vi "Motor Move XYZ-AOL Zstack.vi"(8 "error in (no error)":errorcluster, 9 "Zplane in":i32, 10 "AOL_Globals":T1={"Imaging Protocol"=enum."AOL Z-Stack", "Number of POI"=0, "Number of Miniscans"=0, "Number of Trials"=0, "Number of Cycles "=0, "# Averaged Frames"=0, "Laser power (%)"=0, "Pockels (V)"=0.0, "Acquisition Length (sec)"=0.0, "Fill time (us)"=0.0, "POI Dwell time (us)"=0.0, "Miniscan Dwell time per pixel (us)"=0.0, "PMT 1"=0.0, "PMT 2"=0.0, "Back Apperture (mA)"=200.0, "Frame Size"=0, "Center Frequency"=0.0, "Field of View (um)"=175.0, "Field of View (norm)"=0.0, "DwellTime (us)"=0.0, "Ref Dwell Time (us)"=0.0, "Wavelength (nm)"=0.0, "Zoom"=0.0, "AOL Z"=0.0, "AOL Mode"=enum."Raster", "GridXY"=0.0, "GridZ"=0.0, "TriggerPeriod (sec)"=0.0, "Number of Pixels in Miniscan"=0, "Experiment folder path"=path "", "X centre"=0.0, "Y centre"=0.0, "Angle (degrees)"=0.0, "Angle Xs (degrees)"=0.0, "Angle Ys (degrees)"=0.0, "Plane Mode"=0, "Threshold"=[], "Regenerate Chirps"=FALSE, "Rectangle ROI length (pixels)"=0, "Rectangle ROI height (pixels)"=0, "AOD fill"=4900, "StartupDelay"=0, "Samples Wait after Trigger"=5080, "Slip Cycle"=600000, "Add Cycle"=TRUE, "Functional Mode"=enum."Point", "Z Start"=0.0, "Z Stop"=0.0, "# Planes"=0, "Total Pixels"=0, "Variable Miniscan Pixels"=[], "Use Variable Length"=FALSE, "Use Variable Resolution"=FALSE, "Laser power (%) at Z Start"=0, "Laser power (%) at Z Stop"=0, "Ref Z Step"=0} {"Angle Ys (degrees)" format="%#.6g"; "Angle Xs (degrees)" format="%#.6g"; "Plane Mode" items=["XY Plane", "XZ Plane", "YZ Plane", "arbitraryplane"]; "Frame Size" items=["100X100"=100, "128X128"=128, "200X200"=200, "256X256"=256, "512X512"=512, "1024x1024"=1024, "2048x2048"=2048]; "Back Apperture (mA)" format="%#.6g"; "Pockels (V)" format="%#.6g"; "PMT 2" format="%#.6g"; "PMT 1" format="%#.6g"; "Angle (degrees)" format="%#.6g"; "POI Dwell time (us)" format="%#.6g"}) -> (0 "error out":errorcluster)   [LabVIEW 2020]
uses:
  Typedefs/Controls/AOL_Globals.ctl
  Typedefs/Imaging Protocols enum.ctl
  Typedefs/Frame Size.ctl
  Typedefs/AOL modes.ctl
  Typedefs/Plane Mode.ctl
  Typedefs/Functional Mode.ctl
  Typedefs/HW config states enum.ctl
  Typedefs/Read Write Enum.ctl
  Global Variables/General Globals.vi
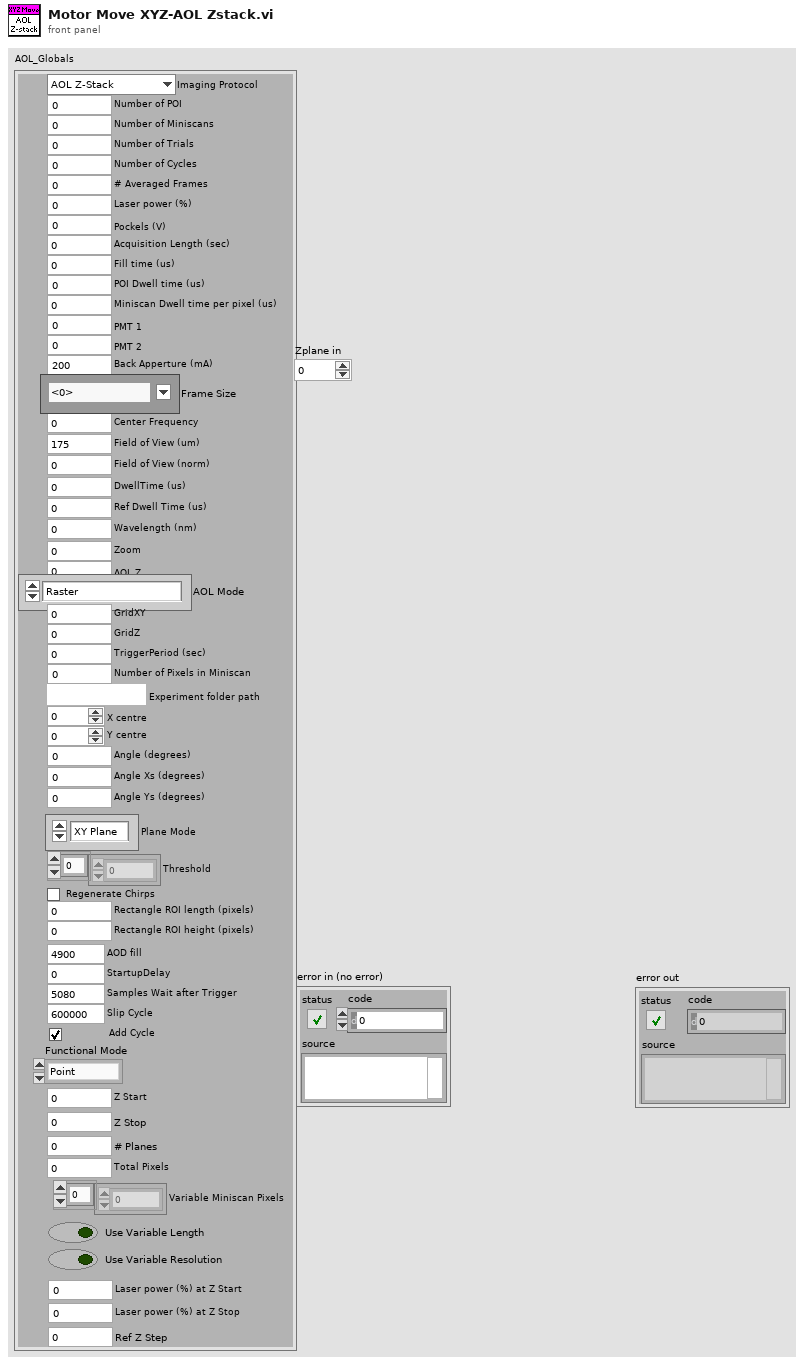
[diagram p1: front panel]
types:
  T1 = typedef "AOL_Globals.ctl" = cluster{"Imaging Protocol":T2, "Number of POI":u16, "Number of Miniscans":u16, "Number of Trials":u16, "Number of Cycles ":u64, "# Averaged Frames":u16, "Laser power (%)":u8, "Pockels (V)":dbl, "Acquisition Length (sec)":dbl, "Fill time (us)":dbl, "POI Dwell time (us)":dbl, "Miniscan Dwell time per pixel (us)":dbl, "PMT 1":dbl, "PMT 2":dbl, "Back Apperture (mA)":dbl, "Frame Size":T3, "Center Frequency":dbl, "Field of View (um)":dbl, "Field of View (norm)":dbl, "DwellTime (us)":dbl, "Ref Dwell Time (us)":dbl, "Wavelength (nm)":dbl, "Zoom":dbl, "AOL Z":dbl, "AOL Mode":T4, "GridXY":dbl, "GridZ":dbl, "TriggerPeriod (sec)":dbl, "Number of Pixels in Miniscan":u16, "Experiment folder path":path, "X centre":dbl, "Y centre":dbl, "Angle (degrees)":dbl, "Angle Xs (degrees)":dbl, "Angle Ys (degrees)":dbl, "Plane Mode":T5, "Threshold":u16[], "Regenerate Chirps":bool, "Rectangle ROI length (pixels)":u16, "Rectangle ROI height (pixels)":u16, "AOD fill":u16, "StartupDelay":i32, "Samples Wait after Trigger":u16, "Slip Cycle":u32, "Add Cycle":bool, "Functional Mode":T6, "Z Start":dbl, "Z Stop":dbl, "# Planes":i32, "Total Pixels":i32, "Variable Miniscan Pixels":u16[], "Use Variable Length":bool, "Use Variable Resolution":bool, "Laser power (%) at Z Start":u8, "Laser power (%) at Z Stop":u8, "Ref Z Step":i8}
  T2 = typedef "Imaging Protocols enum.ctl" = enum16{"AOL Z-Stack", "Motor Z Stack", "Parameter Sweep", "Functional Acquisition", "Single Plane Acquisition", "Volume Acquisition", "Live Imaging", "Live Plane Imaging", "Live Volume Imaging"}
  T3 = typedef "Frame Size.ctl" = u16
  T4 = typedef "AOL modes.ctl" = enum16{"Raster", "Structural", "Pointing", "Mini Scan", "Alignment"}
  T5 = typedef "Plane Mode.ctl" = u16
  T6 = typedef "Functional Mode.ctl" = enum16{"Point", "Line", "Patch", "Plane", "Volume"}
  T7 = typedef "HW config states enum.ctl" = enum16{"Load from file", "Save to file", "Save backup", "Write all", "Read all", "Write XY stage settings", "Write DAQ FPGA settings", "Write Control FPGA settings", "Write Phys Channels", "Write System Config", "Write HW Config", "Save System Config", "Save HW Config", "Clear", "Compare from file"}
  T8 = typedef "Read Write Enum.ctl" = enum16{"Read", "Write"}
  T9 = typedef "Hardware Configuration settings.ctl" = cluster{"Dev. PC":bool, "Swap XY on stage":bool, "No of AOD":u8, "MC Supported":bool, "Axial MC":bool, "Computer MAC address":string, "Externalise Triggers":bool, "Trigger HW config":T10, "DAQmx Chan":T11, "XYZ Stage Control Config":T12, "XY stage available":bool, "XY Comms Config Cluster":T13, "Y stage available":bool, "Y Comms Config Cluster":T13, "Z stage available":bool, "Z Comms Config Cluster ":T13, "Encoder available":bool, "Encoder":T15, "VidRec available":bool, "Cam VidRec":T16, "Laser Power Control HW config":T17, "Laser 1 available":bool, "Laser 1 config cluster":T18, "Prechirper 1 available":bool, "Prechirper 1 config cluster":T19, "Control system.FPGA available?":bool, "Control Sys. HW config":T20, "DAQ FPGA HW Config":T21, "PMT Control Voltage Limits":T25}
  T10 = typedef "Triggers HW config.ctl" = cluster{"Available Device List":i32, "Device Address":string}
  T11 = typedef "DAQmx physical channels cluster.ctl" = cluster{"Pockels AO":tag, "Hard shutter AO":tag, "PMT AOs":tag, "Galvo AOs":tag, "Power meter AI":tag}
  T12 = typedef "XYZControlConfig.ctl" = enum16{"None", "XYZ", "XY-Z", "X-Y-Z", "Z"}
  T13 = typedef "Peripherals comms config cluster.ctl" = cluster{"Name":string, "Device Address":string, "Port ":u16, "Baudrate":i32, "Comms Type":T14}
  T14 = typedef "Comms Type.ctl" = enum16{"GPIB-IEEE488", "Serial-RS232", "Serial-RS485", "Serial-RS422", "Serial-USB", "Ethernet-TCP/IP", "Ethernet-UDP"}
  T15 = typedef "Encoder config cluster.ctl" = cluster{"IP address":string, "Port":u16, "Wheel radius (cm)":dbl, "Encoder Trigger":tag}
  T16 = typedef "Cam VidRec HW config setup cluster.ctl" = cluster{"DO flag-Video record":tag, "DO flag-Trial start":tag}
  T17 = typedef "Laser Power Control HW config.ctl" = cluster{"Laser Power Control":string, "Laser Power Modulation Control":enum16{"NI", "FPGA"}}
  T18 = typedef "Laser 1 config cluster.ctl" = cluster{"COM port":refnum<visa-resource-name>, "Baud Rate":i32, "Type":string}
  T19 = typedef "PreChirper 1 config cluster.ctl" = cluster{"Type":string, "Baud Rate":i32, "COM port":refnum<visa-resource-name>}
  T20 = typedef "Control Sys HW config cluster.ctl" = cluster{"Control system.FPGA Type":enum16{"Virtex 5", "Virtex 7"}, "Control system.Network adapter name":string, "Control system.MAC address":string, "Control system.Ethernet Port":u32, "Control system.Ethernet Port Opened":bool}
  T21 = typedef "DAQ FPGA HW config cluster.ctl" = cluster{"FGPA Ref":T22, "Target":T23, "input card type":T24}
  T22 = typedef "FPGA Ref.ctl" = refnum<k20>
  T23 = typedef "nirio_resource_hc.ctl" = tag
  T24 = typedef "FPGA input type AC-DC.ctl" = enum16{"AC Card", "DC Card"}
  T25 = typedef "PMT Control Voltage limits.ctl" = cluster{"Lower Limit":dbl, "Upper Limit":dbl}
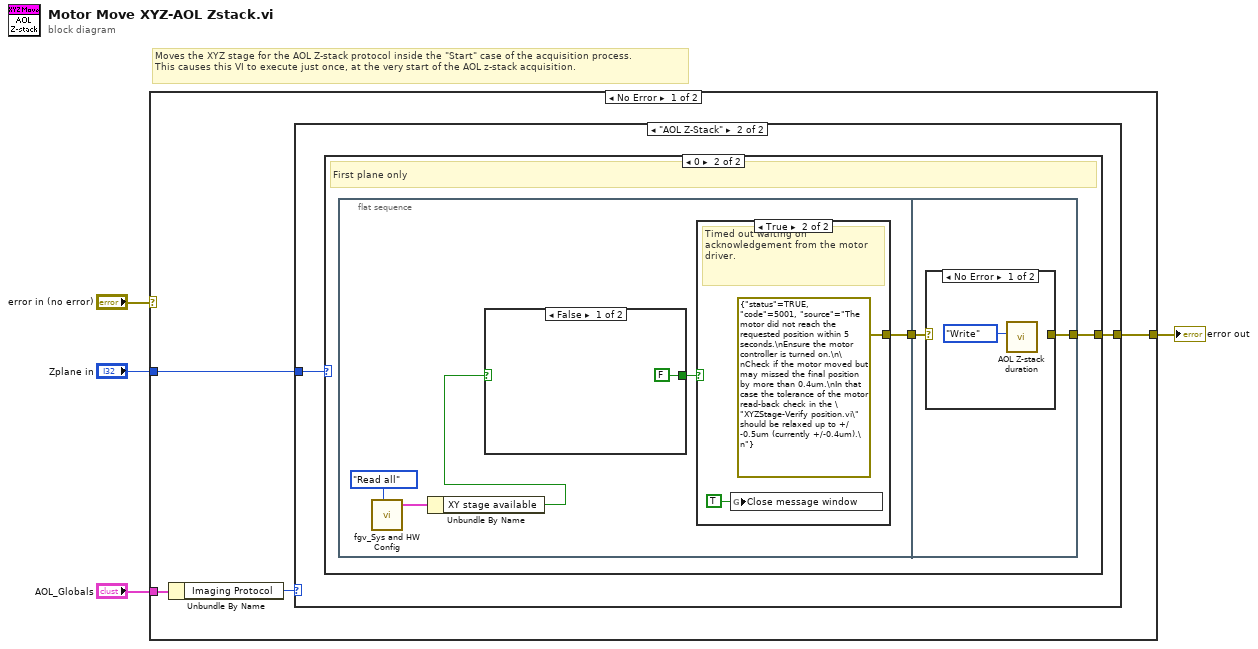
[diagram p0: block diagram]
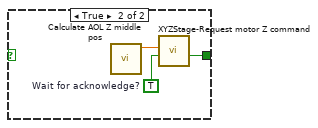
[diagram p4: hidden frame]
diagram:
  # "Moves the XYZ stage for the AOL Z-stack protocol inside the \"Start\" case of the acquisition process.\nThis causes this VI to execute just once, at the very start of the AOL z-stack acquisition."
  n1 = case shown="No Error" "error in (no error)" {
    selector: "error in (no error)" -> [_ w28]
    tunnel: [w5 w28] -> w3
    tunnel: "AOL_Globals" -> [w7 _]
    tunnel: "Zplane in" -> [w6 _]
    frame No Error {
      n2 = Unbundle By Name(w7) -> ("Imaging Protocol"=w8:T2)
      n3 = case shown="\"AOL Z-Stack\"" w8 {
        tunnel: w6 -> [_ w10]
        tunnel: [_ w9] -> w5
        frame Default {
        }
        frame "AOL Z-Stack" {
          n4 = case shown="0" w10 {
            tunnel: [_ w11] -> w9
            frame Default {
            }
            frame 0 {
              # "First plane only"
              n5 = flat-sequence {
                tunnel: [w16] -> w12
                tunnel: w12 -> [w25]
                tunnel: [w24] -> w11
                frame #0 {
                  n6 = call "fgv_Sys and HW Config.vi"("Function"=HW_config_states_enum."Read all") -> ("Hardware Configuration OUT"=w15:T9)  [unwired: 8 in, 2 out]
                  n7 = Unbundle By Name(w15) -> ("XY stage available"=w13:bool)
                  n8 = case shown="False" w13 {
                    tunnel: [FALSE ("Timed out while waiting for acknowledgement") w19] -> w17
                    frame False {
                    }
                    frame True {
                      w20 = TRUE  # Wait for acknowledge?
                      n9 = call "Calculate AOL Z middle pos.vi"() -> ("AOL Z-stack middle position"=w21:dbl)  [unwired: 11 in]
                      n10 = call "XYZStage-Request motor Z command.vi"("Wait for acknowledge?"=w20, "Motor Z"=w21) -> ("Timed out while waiting for acknowledgement"=w19:bool)  [unwired: 7 in, 2 out]
                    }
                  }
                  n11 = case shown="True" w17 {
                    tunnel: [_ errorcluster {"status"=TRUE, "code"=5001, "source"="The motor did not reach the requested position within 5 seconds.\nEnsure the motor controller is turned on.\n\nCheck if the motor moved but may missed the final position by more than 0.4um.\nIn that case the tolerance of the motor read-back check in the \"XYZStage-Verify position.vi\" should be relaxed up to +/-0.5um (currently +/-0.4um).\n"} ("error IO")] -> w16
                    frame False {
                    }
                    frame True {
                      # "Timed out waiting on acknowledgement from the motor driver."
                      n12 = global write "General Globals.vi" "Close message window"(TRUE ("Close message window")) -> ()
                    }
                  }
                }
                frame #1 {
                  n13 = case shown="No Error" w25 {
                    selector: w25 -> [_ w27]
                    tunnel: [_ w27] -> w24
                    frame No Error {
                      n14 = call "AOL Z-stack duration.vi"("Function"=Read_Write_Enum."Write") -> ()  [unwired: 10 in, 1 out]
                    }
                    frame Error {
                    }
                  }
                }
              }
            }
          }
        }
      }
    }
    frame Error {
    }
  }
  "error out" <- w3
